vi "picoquant_initialize_log.vi"(8 "error in (no error)":errorcluster, 10 "data_logger":refnum<class "data_logger.lvclass">, 11 "picoharp in":refnum<class "picoharp.lvclass">) -> (0 "error out":errorcluster, 3 "picoharp out":refnum<class "picoharp.lvclass">)   [LabVIEW 2015, in "picoharp.lvclass"]
uses:
  picoharp.lvclass
  Data Logger Class/data_logger.lvclass
  picoharp.lvclass/picoharp.ctl
  Hydraharp/hdf5_photon_record_logger/hdf5_photon_record_log.lvclass
  Hydraharp/hydraharp_panel/hpanel_acq_modes.ctl
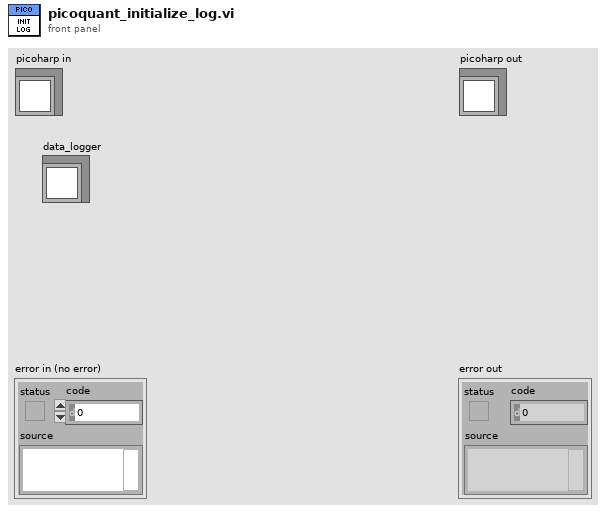
[diagram p1: front panel]
types:
  T1 = typedef "hpanel_acq_modes.ctl" = u16
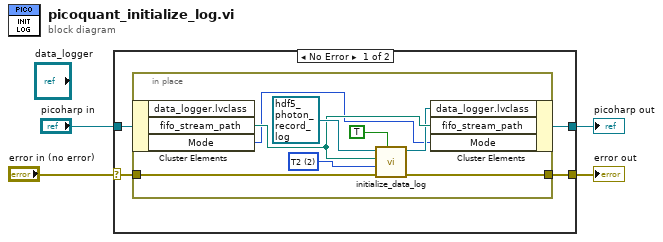
[diagram p0: block diagram]
diagram:
  n1 = case shown="No Error" "error in (no error)" {
    selector: "error in (no error)" -> [w7 w17]
    tunnel: "picoharp in" -> [w8 w18]
    tunnel: [w6 w17] -> w1
    tunnel: [w5 w18] -> w2
    frame No Error {
      n2 = in-place {
        in-place-border: w7 -> [w13]
        in-place-border: [w12] -> w6
        w9 = T1 2 items=["T2"=2, "T3"=3] ("data")
        n3 = in-place-cluster #1(w8) -> ("fifo_stream_path"=w14:path, "Mode"=w10:T1)  [unwired: 1 out]
        n4 = call-dynamic "initialize_data_log.vi"("Overwrite?"=TRUE, "error in (no error)"=w13, "Initialization Data"=w9, "Path"=w14, "hdf5_photon_record_log in"=refnum<class "hdf5_photon_record_log.lvclass"> refnum ("hdf5_photon_record_log.lvclass")) -> ("error out"=w12:errorcluster, "hdf5_photon_record_log out"=w11:refnum<class "hdf5_photon_record_log.lvclass">)  [unwired: 5 in]
        n5 = in-place-cluster #1("data_logger.lvclass"=w11, "fifo_stream_path"=w14, "Mode"=w10) -> (w5:refnum<class "picoharp.lvclass">)
      }
    }
    frame Error {
    }
  }
  "error out" <- w1
  "picoharp out" <- w2
